vi "Edit Program.vi"(8 "Error In":errorcluster, 9 "Program Source":string, 10 "Program Handle":T2, 11 "Device In":T1) -> (0 "Error Out":errorcluster, 2 "Program Handle":T2, 3 "Device Out":T1)   [LabVIEW 2012, in "OpenCLV x64.lvlib"]
doc: "A sub-vi that is only meant to pop-up if there are OpenCL compile errors. Not supposed to be seen or used by the user."
uses:
  OpenCLV x64.lvlib
  Controls/Device ID.ctl
  Controls/Program Handle.ctl
  Error Checking/Add Error Functional Global.vi
panel:
  in  "Open Button":bool
  in  "Cancel Button":bool
  in  "Save As Button":bool
  in  "Compile Button":bool
  in  "Finished":bool
  out "Compile Log":string
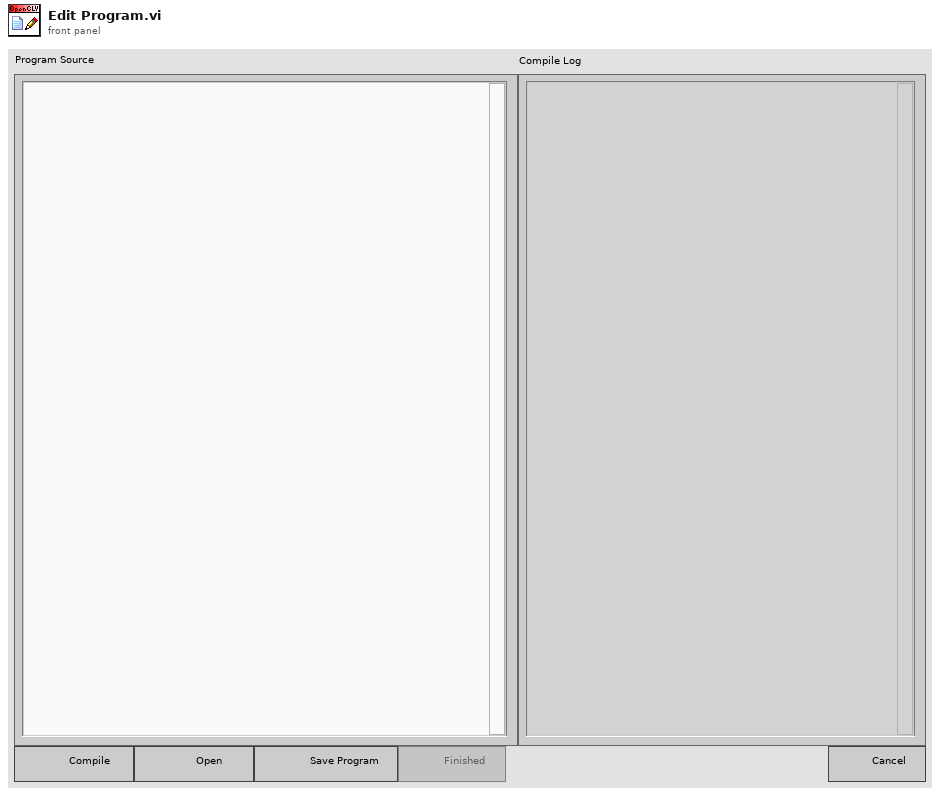
[diagram p1: front panel]
types:
  T1 = typedef "OpenCLV x64.lvlib/Device ID.ctl" = u64
  T2 = typedef "OpenCLV x64.lvlib/Program Handle.ctl" = u64
  T3 = enum8{"Enabled", "Disabled", "Disabled and Grayed Out"}
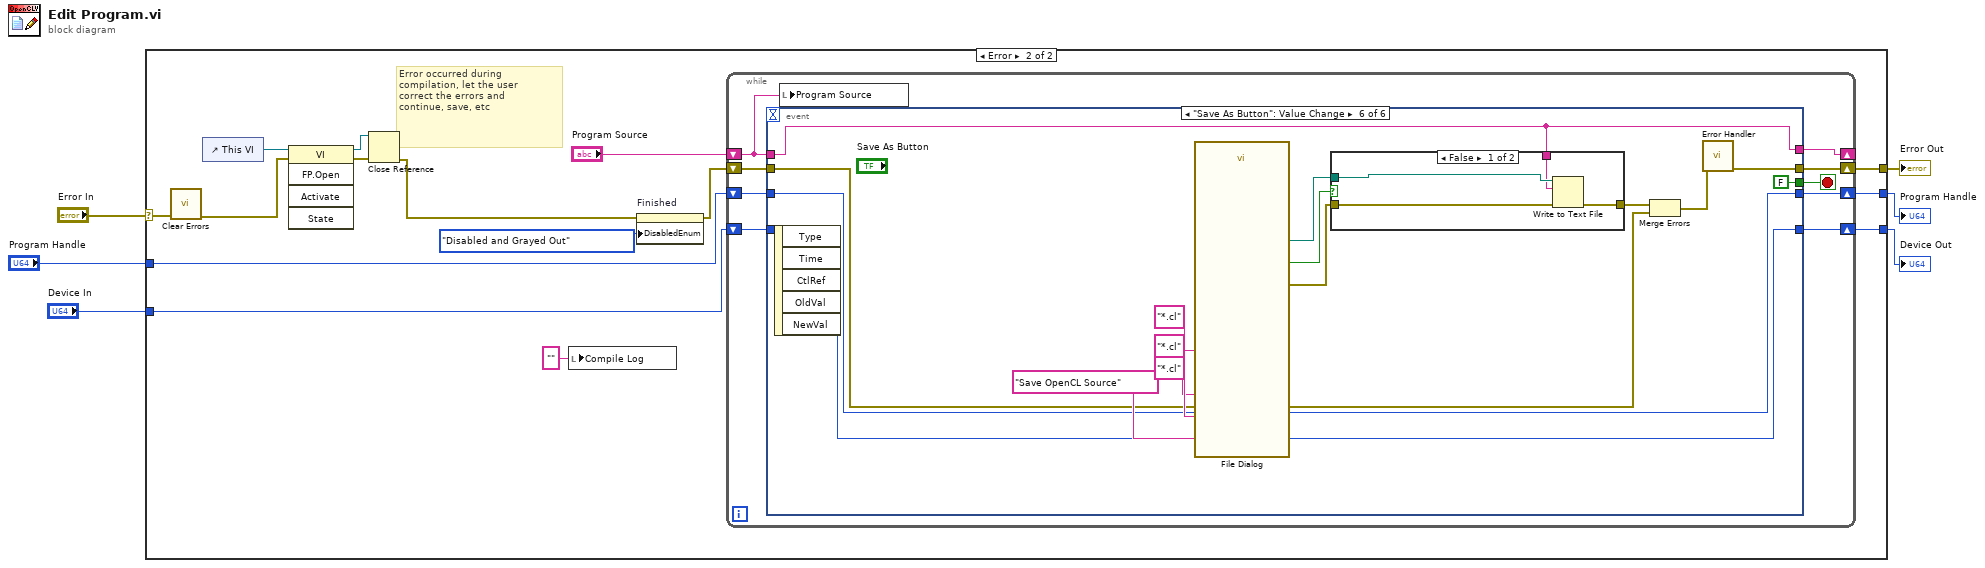
[diagram p0: block diagram]
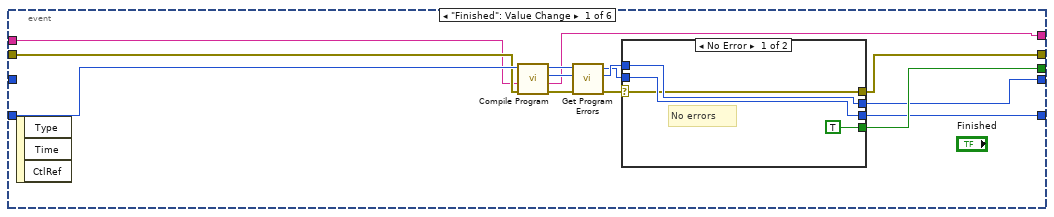
[diagram p3: hidden frame]
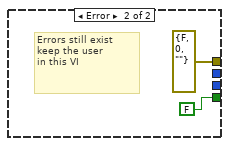
[diagram p4: hidden frame]
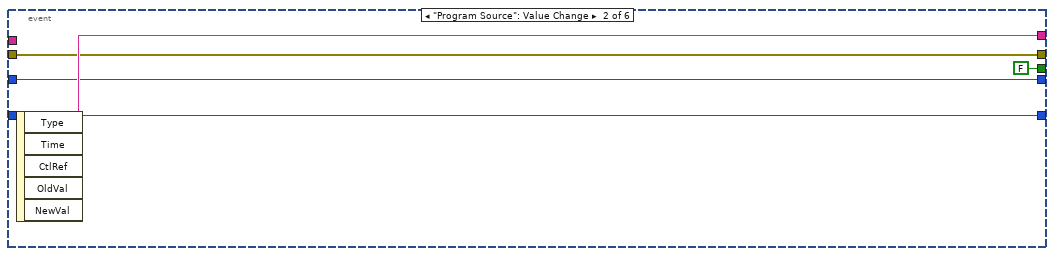
[diagram p5: hidden frame]
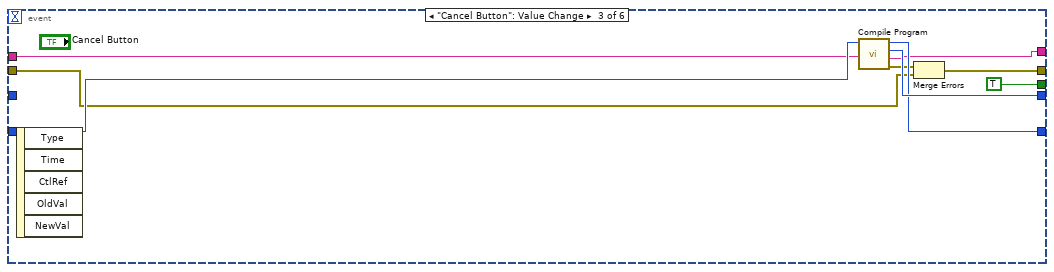
[diagram p6: hidden frame]
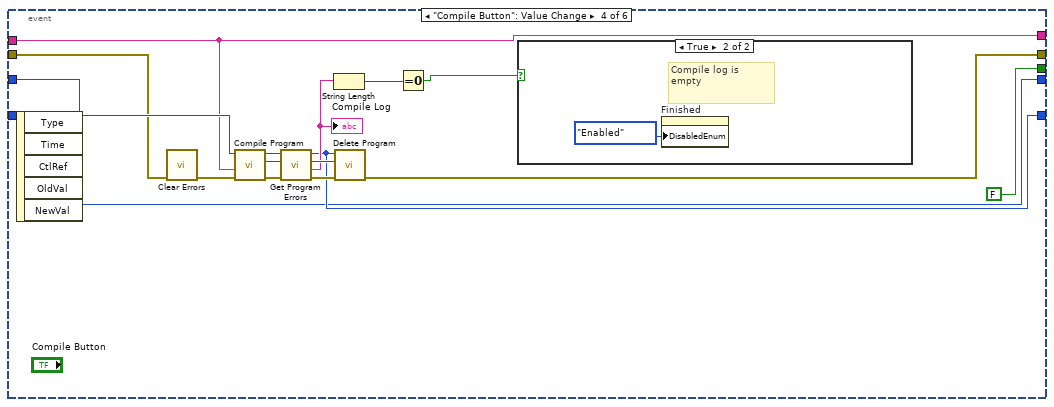
[diagram p7: hidden frame]
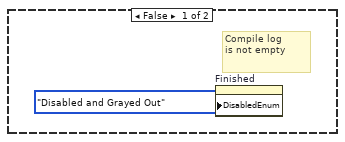
[diagram p8: hidden frame]
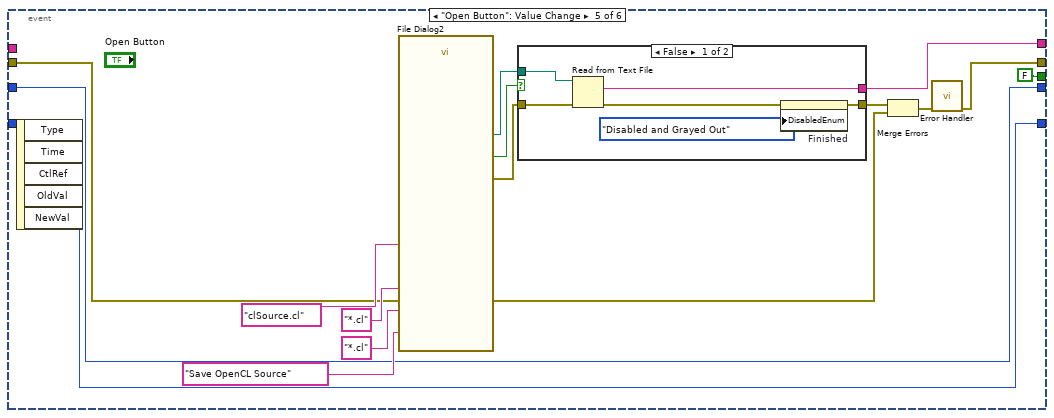
[diagram p9: hidden frame]
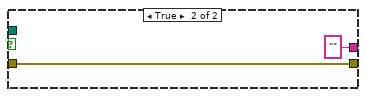
[diagram p10: hidden frame]
diagram:
  n1 = case shown="Error" "Error In" {
    selector: "Error In" -> [w7 w16]
    tunnel: [w7 w22] -> w5
    tunnel: "Program Handle" -> [w8 w20]
    tunnel: "Device In" -> [w9 w21]
    tunnel: [w8 w19] -> w2
    tunnel: [w9 w18] -> w1
    frame No Error {
      # "No error, program has been compiled and is ready to go,\ndon't show the front panel"
    }
    frame Error {
      # "Error occurred during\ncompilation, let the user\ncorrect the errors and \ncontinue, save, etc"
      n2 = call <vilib>:"Clear Errors.vi"("error in (no error)"=w16) -> ("error out"=w13:errorcluster)  [unwired: 6 in]
      n3 = control-ref of="This VI"() -> (w14:refnum<vi>)
      n4 = invoke class="VI" method="FP.Open"(reference=w14, error in=w13) -> (reference out=w11:refnum<vi>, error out=w12:errorcluster)  [unwired: 3 in, 3 out]
      n5 = Close Reference(reference=w11, error in (no error)=w12) -> (error out=w10:errorcluster)
      n6 = local write "Compile Log"("") -> ()
      n7 = property on="Finished" class="Bool"(error in=w10, "DisabledEnum"=T3."Disabled and Grayed Out" ("Disabled")) -> (error out=w23:errorcluster)  [unwired: 1 in, 1 out]
      n8 = while {
        shift-right: [w31] -> w22
        shift-left: w23 -> [w27]
        shift-right: [w29] -> w18
        shift-left: w21 -> [w32]
        shift-right: [w30] -> w19
        shift-left: w20 -> [w28]
        shift-right: [w26] -> _
        shift-left: "Program Source" -> [w25]
        stop <- w33 stop-if-true
        n9 = event shown="[5] \"Save As Button\": Value Change" {
          selector: _ -> [_ _ _ _ _ _]
          dyn-events: _ -> [_ _ _ _ _ _]
          timeout: _ -> [_ _ _ _ _ _]
          tunnel: [w43 FALSE TRUE FALSE FALSE FALSE] -> w33
          tunnel: w32 -> [w45 w55 w66 w83 w93 w116]
          tunnel: [w37 w57 w63 w73 w87 w110] -> w31
          tunnel: [w40 w56 w65 w74 w92 w115] -> w30
          tunnel: [w38 w55 w64 w76 w93 w116] -> w29
          tunnel: w28 -> [_ w56 _ w74 w92 w115]
          tunnel: w27 -> [w36 w57 w61 w68 w89 w113]
          tunnel: w25 -> [w35 _ w60 w72 _ w109]
          tunnel: [w34 w58 w59 w72 w86 w109] -> w26
          event "Finished": Value Change {
            n10 = event-data() -> ()  [unwired: 1 in, 3 out]
            n11 = call "Compile Program.vi"("error in (no error)"=w36, "OpenCL Source Code"=w35, "Device In in"=w45) -> ("error out"=w42:errorcluster, "OpenCL Source Code Out"=w34:string, "Program Handle"=w46:T2, "Device Out"=w47:T1)  [unwired: 5 in]
            n12 = call "Get Program Errors.vi"("Error In"=w42, "Program Handle"=w46, "Device In"=w47) -> ("Error Out"=w41:errorcluster, "Program Out"=w44:T2, "Device Out"=w39:T1)  [unwired: 5 in, 1 out]
            n13 = case shown="No Error" w41 {
              selector: w41 -> [w48 _]
              tunnel: w44 -> [w50 _]
              tunnel: [TRUE FALSE] -> w43
              tunnel: [w50 _] -> w40
              tunnel: [w49 _] -> w38
              tunnel: w39 -> [w49 _]
              tunnel: [w48 errorcluster {"status"=FALSE, "code"=0, "source"=""} ("error IO")] -> w37
              frame No Error {
                # "No errors"
              }
              frame Error {
                # "Errors still exist\nkeep the user\nin this VI"
              }
            }
          }
          event "Program Source": Value Change {
            n14 = event-data() -> ("NewVal"=w58:string)  [unwired: 1 in, 4 out]
          }
          event "Cancel Button": Value Change {
            n15 = event-data() -> ()  [unwired: 1 in, 5 out]
            n16 = call "Compile Program.vi"("OpenCL Source Code"=w60, "Device In in"=w66) -> ("error out"=w62:errorcluster, "OpenCL Source Code Out"=w59:string, "Program Handle"=w65:T2, "Device Out"=w64:T1)  [unwired: 6 in]
            n17 = Merge Errors(w62, w61) -> (w63:errorcluster)
          }
          event "Compile Button": Value Change {
            n18 = event-data() -> ()  [unwired: 1 in, 5 out]
            n19 = call <vilib>:"Clear Errors.vi"("error in (no error)"=w68) -> ("error out"=w69:errorcluster)  [unwired: 6 in]
            n20 = call "Compile Program.vi"("error in (no error)"=w69, "OpenCL Source Code"=w72, "Device In in"=w83) -> ("error out"=w80:errorcluster, "Program Handle"=w81:T2, "Device Out"=w82:T1)  [unwired: 5 in, 1 out]
            n21 = call "Get Program Errors.vi"("Error In"=w80, "Program Handle"=w81, "Device In"=w82) -> ("Error Out"=w78:errorcluster, "Compile Log"=w77:string, "Program Out"=w79:T2, "Device Out"=w76:T1)  [unwired: 5 in]
            "Compile Log" <- w77
            n22 = String Length(string=w77) -> (length=w71:i32)
            n23 = call "Delete Program.vi"("Error In"=w78, "Program In"=w79, "Device ID"=w76) -> ("Error Out"=w73:errorcluster)  [unwired: 8 in]
            n24 = Equal To 0?(x=w71) -> (x = 0?=w70:bool)
            n25 = case shown="True" w70 {
              frame False {
                # "Compile log\nis not empty"
                n26 = property on="Finished" class="Bool"("DisabledEnum"=T3."Disabled and Grayed Out" ("Disabled")) -> ()  [unwired: 2 in, 2 out]
              }
              frame True {
                # "Compile log is \nempty"
                n27 = property on="Finished" class="Bool"("DisabledEnum"=T3."Enabled" ("Disabled")) -> ()  [unwired: 2 in, 2 out]
              }
            }
          }
          event "Open Button": Value Change {
            n28 = event-data() -> ()  [unwired: 1 in, 5 out]
            n29 = call "File Dialog2"("prompt"="Save OpenCL Source", "default name"="clSource.cl", "pattern (all files)"="*.cl" ("pattern label"), "pattern label"="*.cl") -> ("selected path"=w99:path, "cancelled"=w98:bool, "error out"=w100:errorcluster)  [unwired: 8 in, 1 out]
            n30 = case shown="False" w98 {
              tunnel: w99 -> [w106 _]
              tunnel: w100 -> [w105 w108]
              tunnel: [w102 w108] -> w90
              tunnel: [w101 ""] -> w86
              frame False {
                n31 = Read from Text File(file (use dialog)=w106, error in=w105) -> (text=w101:string, error out=w103:errorcluster)  [unwired: 2 in, 2 out]
                n32 = property on="Finished" class="Bool"(error in=w103, "DisabledEnum"=T3."Disabled and Grayed Out" ("Disabled")) -> (error out=w102:errorcluster)  [unwired: 1 in, 1 out]
              }
              frame True {
              }
            }
            n33 = Merge Errors(w90, w89) -> (w88:errorcluster)
            n34 = call-poly "Error Handler.vi"("Error In"=w88) -> ("Error Out"=w87:errorcluster)  [unwired: 10 in]
          }
          event "Save As Button": Value Change {
            n35 = event-data() -> ()  [unwired: 1 in, 5 out]
            n36 = call "File Dialog"("prompt"="Save OpenCL Source", "default name"="*.cl", "pattern (all files)"="*.cl" ("pattern label"), "pattern label"="*.cl") -> ("selected path"=w118:path, "cancelled"=w119:bool, "error out"=w117:errorcluster)  [unwired: 8 in, 1 out]
            n37 = case shown="False" w119 {
              tunnel: w118 -> [w127 _]
              tunnel: w117 -> [w126 w128]
              tunnel: [w125 w128] -> w114
              tunnel: w109 -> [w124 _]
              frame False {
                n38 = Write to Text File(file (use dialog)=w127, text=w124, error in=w126) -> (error out=w125:errorcluster)  [unwired: 1 in, 2 out]
              }
              frame True {
              }
            }
            n39 = Merge Errors(w114, w113) -> (w111:errorcluster)
            n40 = call-poly "Error Handler.vi"("Error In"=w111) -> ("Error Out"=w110:errorcluster)  [unwired: 10 in]
          }
        }
        n41 = local write "Program Source"(w25) -> ()
      }
    }
  }
  "Error Out" <- w5
  "Device Out" <- w1
  "Program Handle" <- w2
